vi "Example - Write and Read Multiline Spreadsheet.vi"(8 "error in (no error)":errorcluster) -> (0 "error out":errorcluster)   [LabVIEW 2014, in "SLL Spreadsheet.lvlib"]
uses:
  SLL Spreadsheet.lvlib
panel:
  out "Verified?":bool
  out "2D String[][] Out":string[][](array[string])
  in  "2D String[][]":string[][](array[string])=[["Normal Cell", "Cell with Multiple Lines", "Cell with quote in it "], ["My String", "Line 1\nLine 2\nLine 3", "He says: \"Hello World!\""], ["Item 1, Item 2", "", ""]]
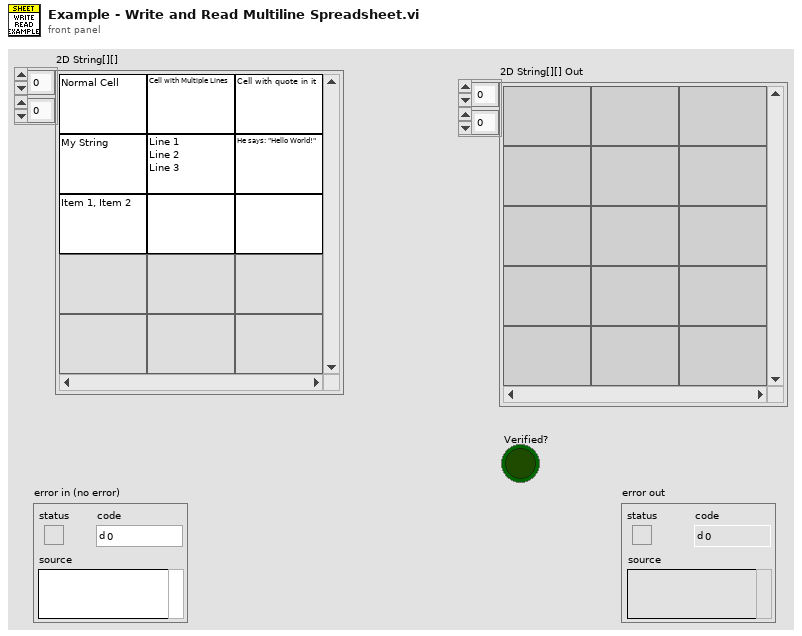
[diagram p1: front panel]
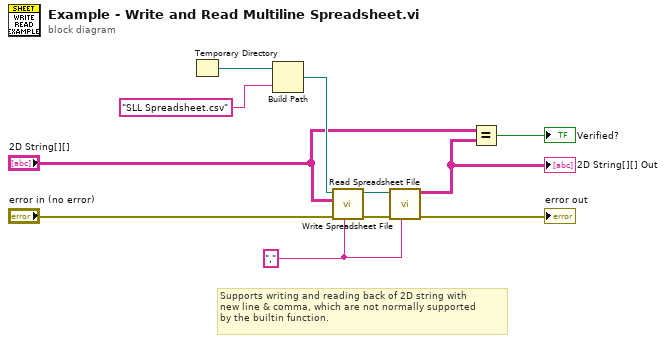
[diagram p0: block diagram]
diagram:
  w5 = "," ("Delimiter (tab)")
  # "Supports writing and reading back of 2D string with\nnew line & comma, which are not normally supported\nby the builtin function."
  n1 = Temporary Directory() -> (w11:path)
  n2 = Build Path(base path=w11, name or relative path="SLL Spreadsheet.csv") -> (appended path=w8:path)
  n3 = call "Write Spreadsheet File.vi"("Delimiter (tab)"=w5, "error in (no error)"="error in (no error)", "2D String[][]"="2D String[][]", "File Path"=w8) -> ("error out"=w7:errorcluster, "File Path dup"=w6:path)  [unwired: 6 in]
  n4 = call "Read Spreadsheet File.vi"("Delimiter (tab)"=w5, "error in (no error)"=w7, "File Path"=w6) -> ("error out"=→"error out":errorcluster, "2D Array"=w3:string[][])  [unwired: 7 in]
  "2D String[][] Out" <- w3
  n5 = Equal?(x="2D String[][]", y=w3) -> (x = y?=→"Verified?":bool)
